vi "Do.vi"(8 "error in (no error)":errorcluster, 10 "Actor in":refnum<class "Actor.lvclass">, 11 "Change Laser Rep Rate":refnum<class "Change Laser Rep Rate.lvclass">) -> (0 "error out":errorcluster, 2 "Actor out":refnum<class "Actor.lvclass">)   [LabVIEW 2014, in "eCRDS Library.lvlib" / "Change Laser Rep Rate.lvclass"]
doc: "(<B>Filename</B>: Actor Framework.lvlib:Message.lvclass:Do.vi)\n\nDefines what a message does when it is received by an actor. Generally, a message instructs an actor to invoke one of its methods. By default, this method does nothing. A child class must override it to define behavior. Create a child class by using the Actor Framework Message Maker dialog box."
uses:
  Change Laser Rep Rate.lvclass
  <vilib>/ActorFramework/Actor/Actor.lvclass
  Change Laser Rep Rate.lvclass/Change Laser Rep Rate.ctl
  Instr Actor/Instr Actor.lvclass
  Commands/Update Laser/Update Laser rate and DC.lvclass
  Commands/Update Laser/Update Laser rate and DC.lvclass/Update Laser rate and DC.ctl
  SuperActor/SuperActor.lvclass/SuperActor.ctl
  SuperActor/Read CVT Session.vi
  SuperActor/Read Log Session.vi
  <userlib>/_Session Fwk/Session - Root.lvclass
  reusable/Command/Command.lvclass
  reusable/Session APIs/CVT/CVT.lvclass
  reusable/Session APIs/Session Log/System Log.lvclass
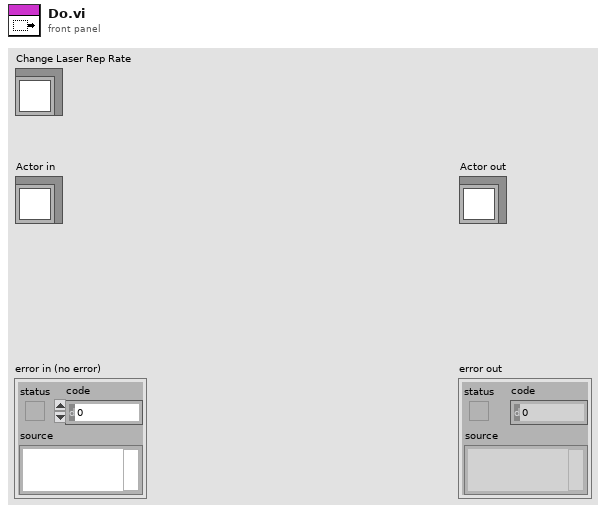
[diagram p1: front panel]
types:
  T1 = typedef "Session - Root.lvclass/Session Handle.ctl" = refnum<data-value>
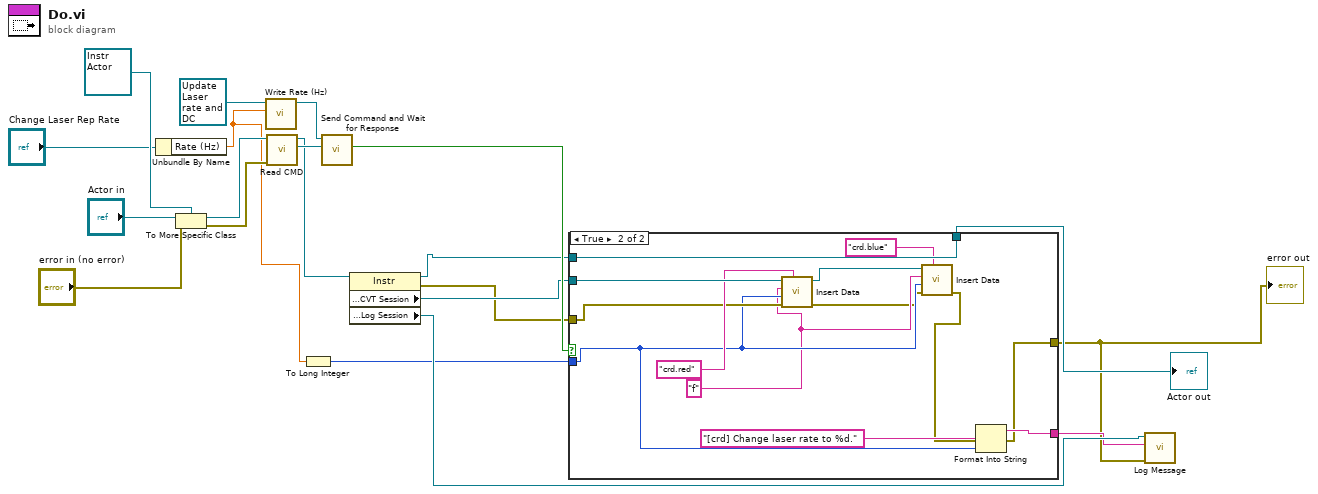
[diagram p0: block diagram]
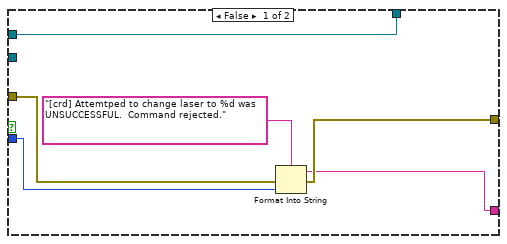
[diagram p2: hidden frame]
diagram:
  n1 = Unbundle By Name("Change Laser Rep Rate") -> ("Rate (Hz)"=w5:dbl)
  n2 = To More Specific Class(target class=refnum<class "Instr Actor.lvclass"> refnum ("Instrument Lib:Instr"), reference="Actor in", error in="error in (no error)") -> (specific class reference=w20:refnum<class "Instr Actor.lvclass">, error out=w19:errorcluster)
  n3 = call "Write Rate (Hz).vi"("Rate (Hz)"=w5, "Update Laser rate and DC in"=refnum<class "Update Laser rate and DC.lvclass"> refnum ("eCRDS Library.lvlib:Update Laser rate and DC.lvclass")) -> ("Update Laser rate and DC out"=w14:refnum<class "Update Laser rate and DC.lvclass">)  [unwired: 8 in, 1 out]
  n4 = call "Read CMD.vi"("error in (no error)"=w19, "Instr Actor in"=w20) -> ("CMD"=w13:refnum<queue>, "Instr Actor out"=w12:refnum<class "Instr Actor.lvclass">)  [unwired: 7 in, 1 out]
  n5 = To Long Integer(number=w5) -> (32bit integer=w1:i32)
  n6 = call "Send Command and Wait for Response.vi"("cmd queue"=w13, "CMD in"=w14) -> ("cmd good?"=w10:bool)  [unwired: 7 in, 2 out]
  n7 = property class="Instr"(reference=w12) -> (reference out=w7:refnum<class "Instr Actor.lvclass">, error out=w8:errorcluster, "Accessors:CVT Session"=w9:T1, "Accessors:Log Session"=w4:T1)  [unwired: 1 in]
  n8 = case shown="True" w10 {
    tunnel: w1 -> [w25 w30]
    tunnel: w7 -> [w26 w39]
    tunnel: [w26 w39] -> w6
    tunnel: w8 -> [w23 w33]
    tunnel: [w22 w36] -> w2
    tunnel: [w21 w37] -> w3
    tunnel: w9 -> [_ w35]
    frame False {
      n9 = Format Into String(format string="[crd] Attemtped to change laser to %d was UNSUCCESSFUL.  Command rejected.", error in=w23, w25) -> (resulting string=w21:string, error out=w22:errorcluster)  [unwired: 1 in]
    }
    frame True {
      w29 = "f" ("tag")
      n10 = call "Insert Data.vi"("Group"="crd.red", "error in"=w33, "Data"=w30, "tag"=w29, "CVT Session In"=w35) -> ("error out"=w28:errorcluster, "CVT Session Out"=w31:T1)  [unwired: 5 in]
      n11 = call "Insert Data.vi"("Group"="crd.blue", "error in"=w28, "Data"=w30, "tag"=w29, "CVT Session In"=w31) -> ("error out"=w27:errorcluster)  [unwired: 5 in, 1 out]
      n12 = Format Into String(format string="[crd] Change laser rate to %d.", error in=w27, w30) -> (resulting string=w37:string, error out=w36:errorcluster)  [unwired: 1 in]
    }
  }
  "error out" <- w2
  "Actor out" <- w6
  n13 = call "Log Message.vi"("error in"=w2, "MSG In"=w3, "session in"=w4) -> ()  [unwired: 7 in, 2 out]
